vi "Transcriptor LabVIEW to C code Translator Native Functions.vi"(0 "Input":variant=variant("Function Name"=variant(string "Strip Path"), "Input Datatypes"=variant(string[] ["error", "int"]), "Inputs"=variant(string[] ["error in", "x"]), "Node refnum"=variant(refnum<vi> refnum), "Output Datatypes"=variant(string[] ["int"]), "Outputs"=variant(string[] ["a"])), 11 "error in (no error)":errorcluster) -> (4 "Output":variant=variant("Defines"=variant(string[] []), "Includes"=variant(string[] []), "Replaced Code"=variant(string "/* LabVIEW system function 'Strip Path' not found. */")), 15 "error out":errorcluster)   [LabVIEW 2014]
doc: "An example of how to create the Translator to convert the LabVIEW VIs to Arduino C code."
panel:
  out "Outputs":string[](array[string])
  out "Inputs":string[](array[string])
  out "Output Datatypes":string[](array[string])
  out "Input Datatypes":string[](array[string])
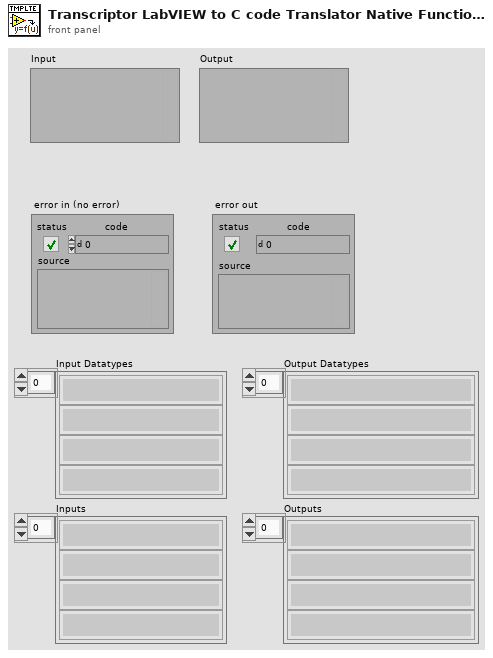
[diagram p1: front panel]
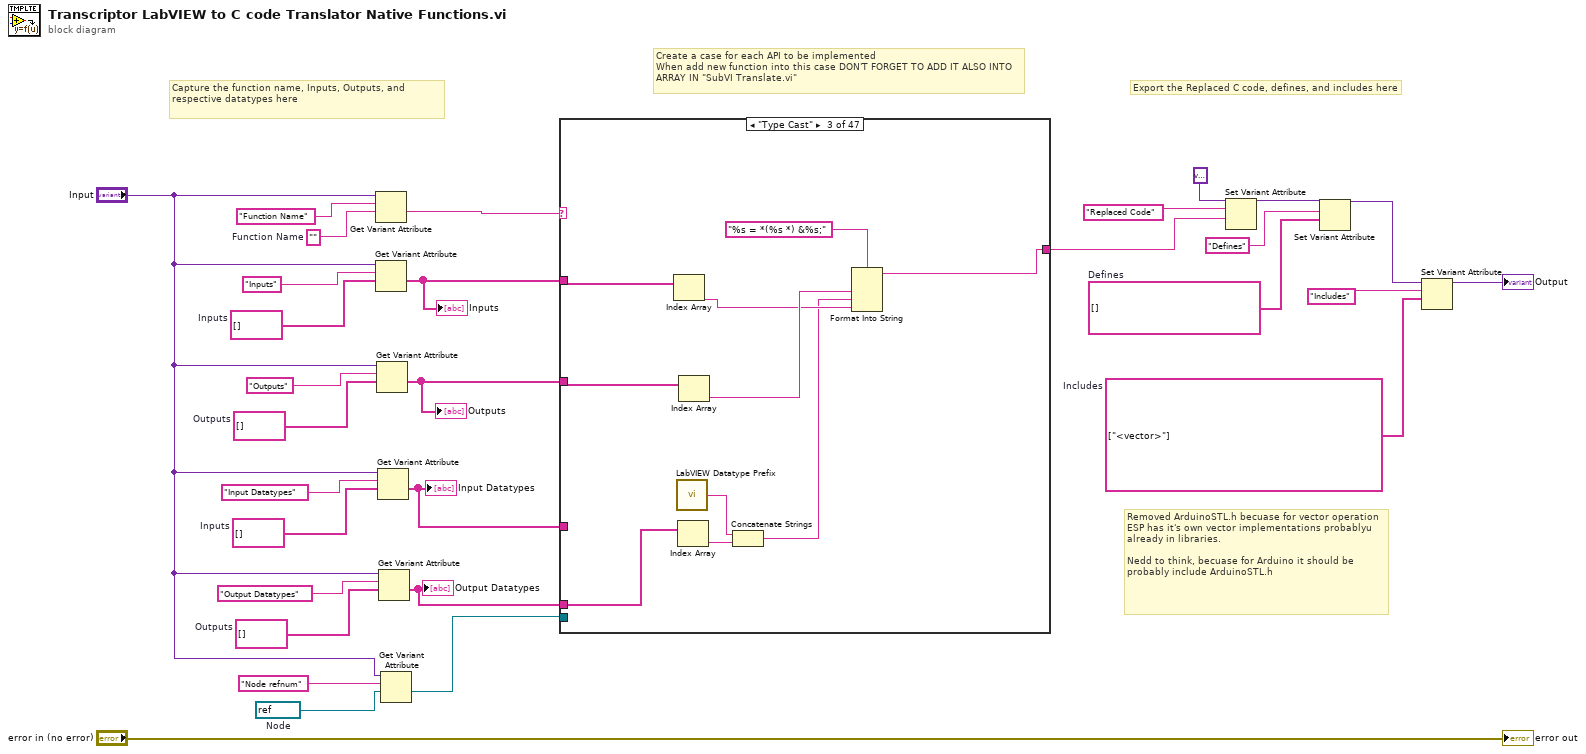
[diagram p0: block diagram]
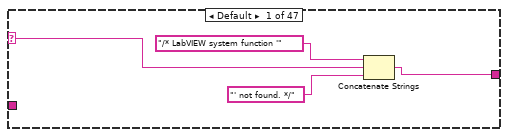
[diagram p2: hidden frame]
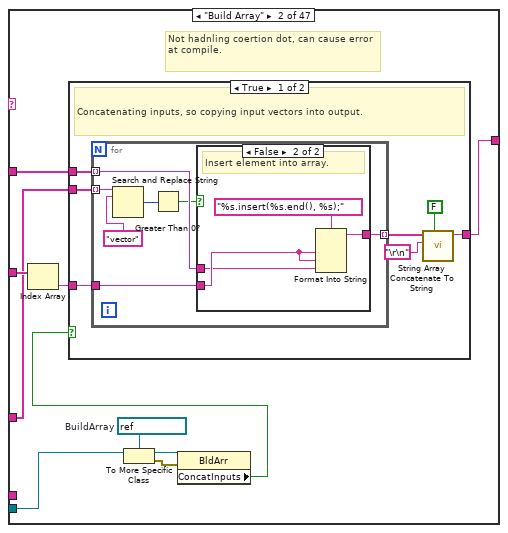
[diagram p3: hidden frame]
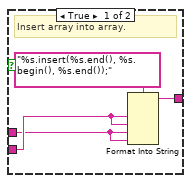
[diagram p4: hidden frame]
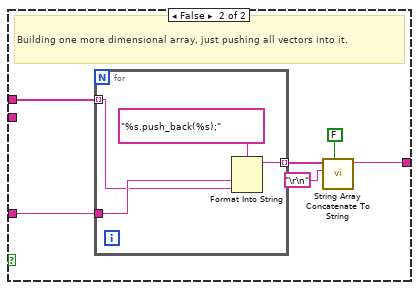
[diagram p5: hidden frame]
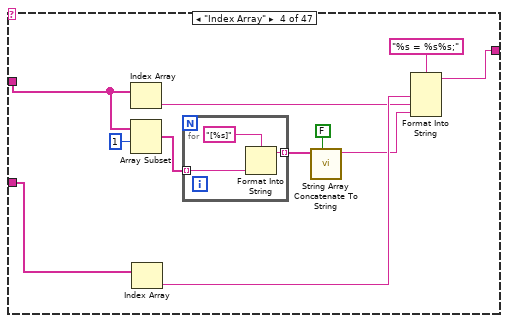
[diagram p6: hidden frame]
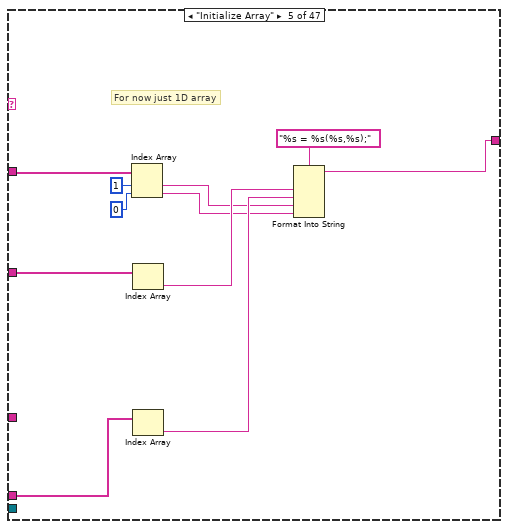
[diagram p7: hidden frame]
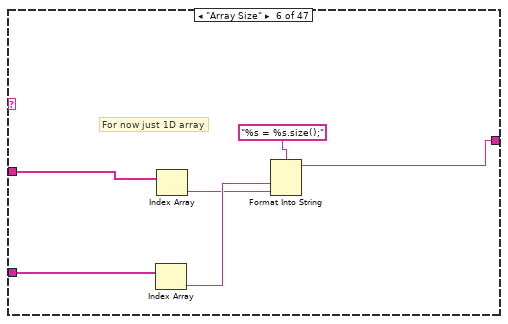
[diagram p8: hidden frame]
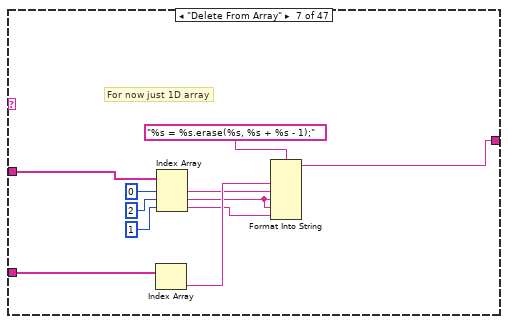
[diagram p9: hidden frame]
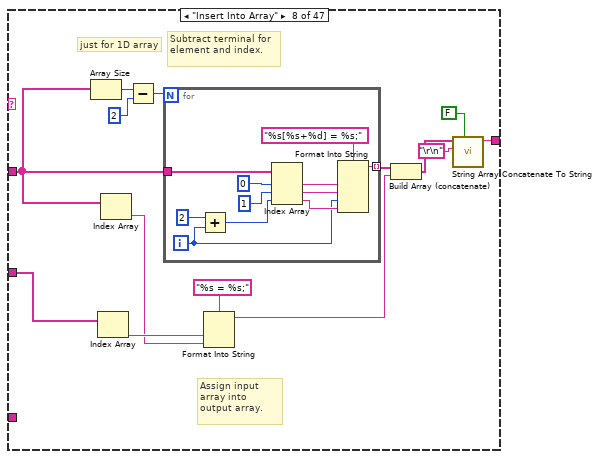
[diagram p10: hidden frame]
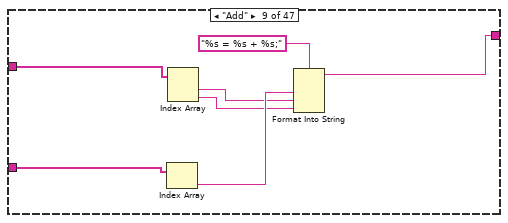
[diagram p11: hidden frame]
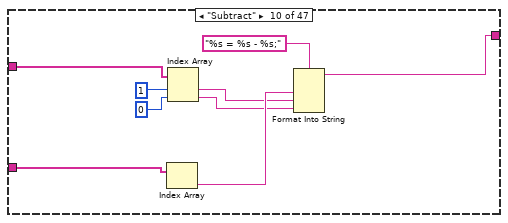
[diagram p12: hidden frame]
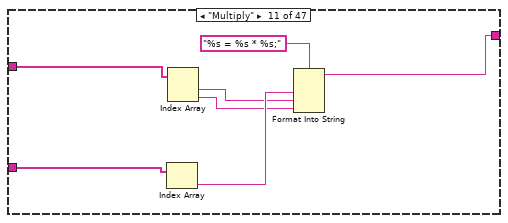
[diagram p13: hidden frame]
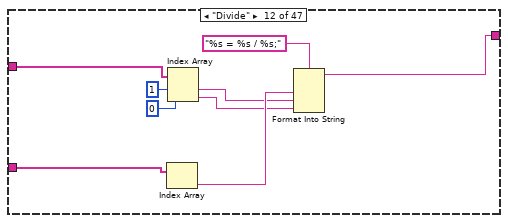
[diagram p14: hidden frame]
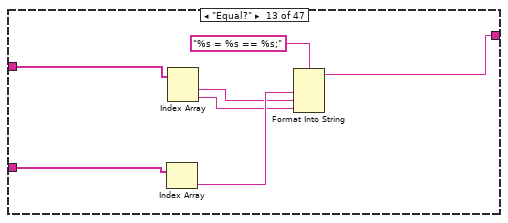
[diagram p15: hidden frame]
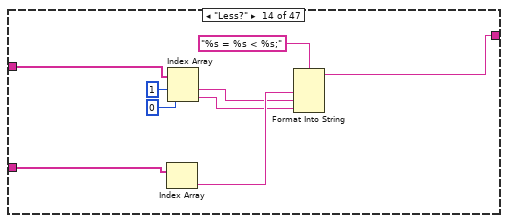
[diagram p16: hidden frame]
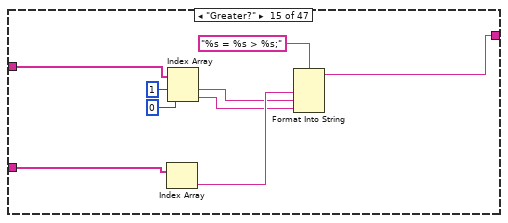
[diagram p17: hidden frame]
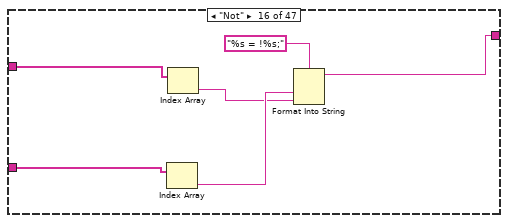
[diagram p18: hidden frame]
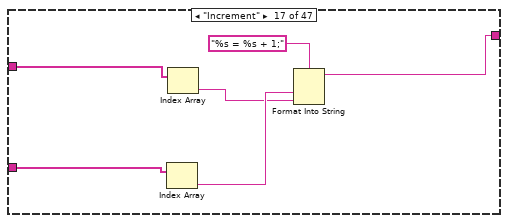
[diagram p19: hidden frame]
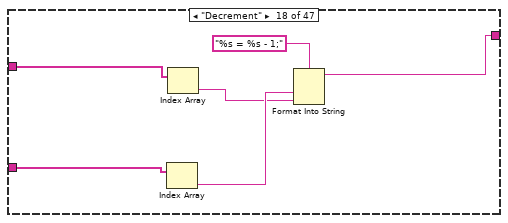
[diagram p20: hidden frame]
diagram:
  w3 = refnum<vi> refnum  # Node
  w7 = string[] []  # Defines
  w15 = string[] []  # Outputs
  w16 = string[] []  # Inputs
  w21 = string[] ["<vector>"]  # Includes
  w26 = string[] []  # Outputs
  w27 = string[] []  # Inputs
  w28 = ""  # Function Name
  # "Removed ArduinoSTL.h becuase for vector operation ESP has it's own vector implementations probablyu already in libraries.\n\nNedd to think, becuase for Arduino it should be probably include ArduinoSTL.h"
  # "Capture the function name, Inputs, Outputs, and respective datatypes here"
  # "Export the Replaced C code, defines, and includes here"
  # "Create a case for each API to be implemented\nWhen add new function into this case DON'T FORGET TO ADD IT ALSO INTO ARRAY IN \"SubVI Translate.vi\""
  n1 = Get Variant Attribute(Variant="Input", name="Function Name", default value (empty Variant)=w28) -> (value=w23:string)  [unwired: 1 in, 3 out]
  n2 = Get Variant Attribute(Variant="Input", name="Inputs", default value (empty Variant)=w27) -> (value=w12:string[])  [unwired: 1 in, 3 out]
  "Inputs" <- w12
  n3 = Get Variant Attribute(Variant="Input", name="Outputs", default value (empty Variant)=w26) -> (value=w13:string[])  [unwired: 1 in, 3 out]
  "Outputs" <- w13
  n4 = Get Variant Attribute(Variant="Input", name="Input Datatypes", default value (empty Variant)=w16) -> (value=w6:string[])  [unwired: 1 in, 3 out]
  "Input Datatypes" <- w6
  n5 = Get Variant Attribute(Variant="Input", name="Output Datatypes", default value (empty Variant)=w15) -> (value=w1:string[])  [unwired: 1 in, 3 out]
  "Output Datatypes" <- w1
  n6 = Get Variant Attribute(Variant="Input", name="Node refnum", default value (empty Variant)=w3) -> (value=w2:refnum<vi>)  [unwired: 1 in, 3 out]
  n7 = case shown="\"Type Cast\"" w23 {
    selector: w23 -> [w33 _ _ _ _ _ _ _ _ _ _ _ _ _ _ _ _ _ _ _ _ _ _ _ _ _ _ _ _ _ _ _ _ _ _ _ _ _ _ _ _ _ _ _ _ _ _]
    tunnel: [w31 w41 w85 w93 w101 w112 w123 w140 w154 w163 w170 w179 w186 w195 w204 w211 w217 w223 w229 w235 w241 w247 w253 w259 w266 w273 w280 w286 w293 w300 w307 w311 w318 w323 w338 w355 w365 w375 w385 w391 w397 w403 w409 w415 w421 w427 w433] -> w22
    tunnel: w12 -> [_ w43 w84 w92 w111 w117 w128 w133 w160 w169 w176 w185 w192 w201 w210 w216 w222 w228 w234 w240 w246 w252 w258 w265 w272 w279 w285 w292 w299 w306 w310 w314 w320 w322 w340 w352 w362 w372 w384 w390 w396 w402 w408 w414 w420 w426 w432]
    tunnel: w13 -> [_ w44 w83 w97 w110 w115 w126 w136 w158 w167 w174 w183 w190 w199 w208 w214 w220 w226 w232 w238 w244 w250 w256 w263 w270 w277 w283 w290 w297 w304 _ _ w316 w321 w339 w349 w359 w369 w380 w389 w395 w401 w407 w413 w419 w425 w431]
    tunnel: w6 -> [_ w35 _ _ _ _ _ _ _ _ _ _ _ _ _ _ _ _ _ _ _ _ _ _ _ _ _ _ _ _ _ _ _ _ _ _ _ _ _ _ _ _ _ _ _ _ _]
    tunnel: w2 -> [_ w40 _ _ _ _ _ _ _ _ _ _ _ _ _ _ _ _ _ _ _ _ _ _ _ _ _ _ _ _ _ _ _ _ _ _ _ _ _ _ _ _ _ _ _ _ _]
    tunnel: w1 -> [_ _ w77 _ w106 _ _ _ _ _ _ _ _ _ _ _ _ _ _ _ _ _ _ _ _ _ _ _ _ _ _ _ _ _ _ _ _ _ _ _ _ _ _ _ _ _ _]
    frame Default {
      n8 = Concatenate Strings("/* LabVIEW system function '", w33, "' not found. */") -> (w31:string)
    }
    frame "Build Array" {
      w39 = refnum<vi> refnum  # BuildArray
      # "Not hadnling coertion dot, can cause error at compile."
      n9 = Index Array(array=w44) -> (element=w42:string)  [unwired: 1 in]
      n10 = To More Specific Class(target class=w39, reference=w40) -> (specific class reference=w38:refnum<vi>, error out=w37:errorcluster)  [unwired: 1 in]
      n11 = property class="BldArr"(reference=w38, error in=w37) -> ("ConcatInputs"=w36:bool)  [unwired: 2 out]
      n12 = case shown="True" w36 {
        tunnel: w43 -> [w51 w72]
        tunnel: w42 -> [w50 w71]
        tunnel: [w46 w67] -> w41
        tunnel: w35 -> [w45 _]
        frame True {
          # "Concatenating inputs, so copying input vectors into output."
          n13 = for {
            tunnel: w51 -> [w57] mode=indexing
            tunnel: w50 -> [w58]
            tunnel: [w56] -> w49 mode=indexing
            tunnel: w45 -> [w55] mode=indexing
            n14 = Search and Replace String(input string=w55, search string="vector" ("name")) -> (number of replacements=w53:i32)  [unwired: 6 in, 3 out]
            n15 = Greater Than 0?(x=w53) -> (x > 0?=w52:bool)
            n16 = case shown="False" w52 {
              tunnel: w58 -> [w61 w65]
              tunnel: w57 -> [w60 w64]
              tunnel: [w59 w63] -> w56
              frame True {
                # "Insert array into array."
                n17 = Format Into String(format string="%s.insert(%s.end(), %s.begin(), %s.end());" ("name"), w61, w61, w60, w60) -> (resulting string=w59:string)  [unwired: 2 in, 1 out]
              }
              frame False {
                # "Insert element into array."
                n18 = Format Into String(format string="%s.insert(%s.end(), %s);" ("name"), w65, w65, w64) -> (resulting string=w63:string)  [unwired: 2 in, 1 out]
              }
            }
          }
          n19 = call "String Array Concatenate To String.vi"("insert last delimiter?"=FALSE, "Delimiter char"="\r\n", "Array String In"=w49) -> ("String"=w46:string)  [unwired: 8 in]
        }
        frame False {
          # "Building one more dimensional array, just pushing all vectors into it."
          n20 = for {
            tunnel: w72 -> [w74] mode=indexing
            tunnel: w71 -> [w75]
            tunnel: [w73] -> w70 mode=indexing
            n21 = Format Into String(format string="%s.push_back(%s);" ("name"), w75, w74) -> (resulting string=w73:string)  [unwired: 2 in, 1 out]
          }
          n22 = call "String Array Concatenate To String.vi"("insert last delimiter?"=FALSE, "Delimiter char"="\r\n", "Array String In"=w70) -> ("String"=w67:string)  [unwired: 8 in]
        }
      }
    }
    frame "Type Cast" {
      n23 = Index Array(array=w84) -> (element=w81:string)  [unwired: 1 in]
      n24 = call "LabVIEW Datatype Prefix.vi"() -> ("datatype prefix"=w78:string)
      n25 = Index Array(array=w77) -> (element=w80:string)  [unwired: 1 in]
      n26 = Index Array(array=w83) -> (element=w82:string)  [unwired: 1 in]
      n27 = Concatenate Strings(w78, w80) -> (w79:string)
      n28 = Format Into String(format string="%s = *(%s *) &%s;" ("name"), w82, w79, w81) -> (resulting string=w85:string)  [unwired: 2 in, 1 out]
    }
    frame "Index Array" {
      n29 = Index Array(array=w92) -> (element=w94:string)  [unwired: 1 in]
      n30 = Array Subset(array=w92, index=1) -> (w90:string[])  [unwired: 1 in]
      n31 = Index Array(array=w97) -> (element=w95:string)  [unwired: 1 in]
      n32 = for {
        tunnel: w90 -> [w99] mode=indexing
        tunnel: [w98] -> w88 mode=indexing
        n33 = Format Into String(format string="[%s]", w99) -> (resulting string=w98:string)  [unwired: 2 in, 1 out]
      }
      n34 = call "String Array Concatenate To String.vi"("insert last delimiter?"=FALSE, "Array String In"=w88) -> ("String"=w87:string)  [unwired: 9 in]
      n35 = Format Into String(format string="%s = %s%s;", w95, w94, w87) -> (resulting string=w93:string)  [unwired: 2 in, 1 out]
    }
    frame "Initialize Array" {
      # "For now just 1D array"
      n36 = Index Array(array=w111, index #1=1 ("index"), index #2=0 ("index")) -> (element #1=w103:string, element #2=w102:string)
      n37 = Index Array(array=w110) -> (element=w108:string)  [unwired: 1 in]
      n38 = Index Array(array=w106) -> (element=w107:string)  [unwired: 1 in]
      n39 = Format Into String(format string="%s = %s(%s,%s);", w108, w107, w103, w102) -> (resulting string=w101:string)  [unwired: 2 in, 1 out]
    }
    frame "Array Size" {
      # "For now just 1D array"
      n40 = Index Array(array=w115) -> (element=w114:string)  [unwired: 1 in]
      n41 = Index Array(array=w117) -> (element=w113:string)  [unwired: 1 in]
      n42 = Format Into String(format string="%s = %s.size();", w114, w113) -> (resulting string=w112:string)  [unwired: 2 in, 1 out]
    }
    frame "Delete From Array" {
      # "For now just 1D array"
      n43 = Index Array(array=w126) -> (element=w125:string)  [unwired: 1 in]
      n44 = Index Array(array=w128, index #1=0 ("index"), index #2=2 ("index"), index #3=1 ("index")) -> (element #1=w124:string, element #2=w119:string, element #3=w118:string)
      n45 = Format Into String(format string="%s = %s.erase(%s, %s + %s - 1);", w125, w124, w119, w119, w118) -> (resulting string=w123:string)  [unwired: 2 in, 1 out]
    }
    frame "Insert Into Array" {
      # "just for 1D array"
      # "Subtract terminal for element and index."
      # "Assign input array into output array."
      n46 = Array Size(array=w133) -> (size(s)=w138:i32)
      n47 = Index Array(array=w136) -> (element=w134:string)  [unwired: 1 in]
      n48 = Index Array(array=w133) -> (element=w132:string)  [unwired: 1 in]
      n49 = Subtract(x=w138, y=2) -> (x-y=w139:i32)
      n50 = for {
        N: w139 -> [_]
        tunnel: w133 -> [w150]
        tunnel: [w151] -> w131 mode=indexing
        i -> [w146]
        n51 = Add(x=2, y=w146) -> (x+y=w145:i32)
        n52 = Index Array(array=w150, index #1=0 ("index"), index #2=1 ("index"), index #3=w145) -> (element #1=w143:string, element #2=w152:string, element #3=w148:string)
        n53 = Format Into String(format string="%s[%s+%d] = %s;", w143, w152, w146, w148) -> (resulting string=w151:string)  [unwired: 2 in, 1 out]
      }
      n54 = Format Into String(format string="%s = %s;", w134, w132) -> (resulting string=w130:string)  [unwired: 2 in, 1 out]
      n55 = Build Array (concatenate)(w131, w130) -> (w129:string[])
      n56 = call "String Array Concatenate To String.vi"("insert last delimiter?"=FALSE, "Delimiter char"="\r\n", "Array String In"=w129) -> ("String"=w140:string)  [unwired: 8 in]
    }
    frame "Add" {
      n57 = Index Array(array=w158) -> (element=w157:string)  [unwired: 1 in]
      n58 = Index Array(array=w160) -> (element #1=w156:string, element #2=w155:string)  [unwired: 2 in]
      n59 = Format Into String(format string="%s = %s + %s;", w157, w156, w155) -> (resulting string=w154:string)  [unwired: 2 in, 1 out]
    }
    frame "Subtract" {
      n60 = Index Array(array=w167) -> (element=w166:string)  [unwired: 1 in]
      n61 = Index Array(array=w169, index #1=1 ("index"), index #2=0 ("index")) -> (element #1=w165:string, element #2=w164:string)
      n62 = Format Into String(format string="%s = %s - %s;", w166, w165, w164) -> (resulting string=w163:string)  [unwired: 2 in, 1 out]
    }
    frame "Multiply" {
      n63 = Index Array(array=w174) -> (element=w173:string)  [unwired: 1 in]
      n64 = Index Array(array=w176) -> (element #1=w172:string, element #2=w171:string)  [unwired: 2 in]
      n65 = Format Into String(format string="%s = %s * %s;", w173, w172, w171) -> (resulting string=w170:string)  [unwired: 2 in, 1 out]
    }
    frame "Divide" {
      n66 = Index Array(array=w183) -> (element=w182:string)  [unwired: 1 in]
      n67 = Index Array(array=w185, index #1=1 ("index"), index #2=0 ("index")) -> (element #1=w181:string, element #2=w180:string)
      n68 = Format Into String(format string="%s = %s / %s;", w182, w181, w180) -> (resulting string=w179:string)  [unwired: 2 in, 1 out]
    }
    frame "Equal?" {
      n69 = Index Array(array=w190) -> (element=w189:string)  [unwired: 1 in]
      n70 = Index Array(array=w192) -> (element #1=w188:string, element #2=w187:string)  [unwired: 2 in]
      n71 = Format Into String(format string="%s = %s == %s;", w189, w188, w187) -> (resulting string=w186:string)  [unwired: 2 in, 1 out]
    }
    frame "Less?" {
      n72 = Index Array(array=w199) -> (element=w198:string)  [unwired: 1 in]
      n73 = Index Array(array=w201, index #1=1 ("index"), index #2=0 ("index")) -> (element #1=w197:string, element #2=w196:string)
      n74 = Format Into String(format string="%s = %s < %s;", w198, w197, w196) -> (resulting string=w195:string)  [unwired: 2 in, 1 out]
    }
    frame "Greater?" {
      n75 = Index Array(array=w208) -> (element=w207:string)  [unwired: 1 in]
      n76 = Index Array(array=w210, index #1=1 ("index"), index #2=0 ("index")) -> (element #1=w206:string, element #2=w205:string)
      n77 = Format Into String(format string="%s = %s > %s;", w207, w206, w205) -> (resulting string=w204:string)  [unwired: 2 in, 1 out]
    }
    frame "Not" {
      n78 = Index Array(array=w214) -> (element=w213:string)  [unwired: 1 in]
      n79 = Index Array(array=w216) -> (element=w212:string)  [unwired: 1 in]
      n80 = Format Into String(format string="%s = !%s;", w213, w212) -> (resulting string=w211:string)  [unwired: 2 in, 1 out]
    }
    frame "Increment" {
      n81 = Index Array(array=w220) -> (element=w219:string)  [unwired: 1 in]
      n82 = Index Array(array=w222) -> (element=w218:string)  [unwired: 1 in]
      n83 = Format Into String(format string="%s = %s + 1;", w219, w218) -> (resulting string=w217:string)  [unwired: 2 in, 1 out]
    }
    frame "Decrement" {
      n84 = Index Array(array=w226) -> (element=w225:string)  [unwired: 1 in]
      n85 = Index Array(array=w228) -> (element=w224:string)  [unwired: 1 in]
      n86 = Format Into String(format string="%s = %s - 1;", w225, w224) -> (resulting string=w223:string)  [unwired: 2 in, 1 out]
    }
    frame "Equal To 0?" {
      n87 = Index Array(array=w232) -> (element=w231:string)  [unwired: 1 in]
      n88 = Index Array(array=w234) -> (element=w230:string)  [unwired: 1 in]
      n89 = Format Into String(format string="%s = (%s == 0);", w231, w230) -> (resulting string=w229:string)  [unwired: 2 in, 1 out]
    }
    frame "Greater Than 0?" {
      n90 = Index Array(array=w238) -> (element=w237:string)  [unwired: 1 in]
      n91 = Index Array(array=w240) -> (element=w236:string)  [unwired: 1 in]
      n92 = Format Into String(format string="%s = (%s > 0);", w237, w236) -> (resulting string=w235:string)  [unwired: 2 in, 1 out]
    }
    frame "Less Than 0?" {
      n93 = Index Array(array=w244) -> (element=w243:string)  [unwired: 1 in]
      n94 = Index Array(array=w246) -> (element=w242:string)  [unwired: 1 in]
      n95 = Format Into String(format string="%s = (%s < 0);", w243, w242) -> (resulting string=w241:string)  [unwired: 2 in, 1 out]
    }
    frame "Greater Or Equal To 0?" {
      n96 = Index Array(array=w250) -> (element=w249:string)  [unwired: 1 in]
      n97 = Index Array(array=w252) -> (element=w248:string)  [unwired: 1 in]
      n98 = Format Into String(format string="%s = (%s >= 0);", w249, w248) -> (resulting string=w247:string)  [unwired: 2 in, 1 out]
    }
    frame "Less Or Equal To 0?" {
      n99 = Index Array(array=w256) -> (element=w255:string)  [unwired: 1 in]
      n100 = Index Array(array=w258) -> (element=w254:string)  [unwired: 1 in]
      n101 = Format Into String(format string="%s = (%s <= 0);", w255, w254) -> (resulting string=w253:string)  [unwired: 2 in, 1 out]
    }
    frame "Greater Or Equal?" {
      n102 = Index Array(array=w263) -> (element=w262:string)  [unwired: 1 in]
      n103 = Index Array(array=w265) -> (element #1=w261:string, element #2=w260:string)  [unwired: 2 in]
      n104 = Format Into String(format string="%s = (%s >= %s);", w262, w261, w260) -> (resulting string=w259:string)  [unwired: 2 in, 1 out]
    }
    frame "Less Or Equal?" {
      n105 = Index Array(array=w270) -> (element=w269:string)  [unwired: 1 in]
      n106 = Index Array(array=w272) -> (element #1=w268:string, element #2=w267:string)  [unwired: 2 in]
      n107 = Format Into String(format string="%s = (%s <= %s);", w269, w268, w267) -> (resulting string=w266:string)  [unwired: 2 in, 1 out]
    }
    frame "Not Equal?" {
      n108 = Index Array(array=w277) -> (element=w276:string)  [unwired: 1 in]
      n109 = Index Array(array=w279) -> (element #1=w275:string, element #2=w274:string)  [unwired: 2 in]
      n110 = Format Into String(format string="%s = (%s != %s);", w276, w275, w274) -> (resulting string=w273:string)  [unwired: 2 in, 1 out]
    }
    frame "Not Equal To 0?" {
      n111 = Index Array(array=w283) -> (element=w282:string)  [unwired: 1 in]
      n112 = Index Array(array=w285) -> (element=w281:string)  [unwired: 1 in]
      n113 = Format Into String(format string="%s = (%s != 0);", w282, w281) -> (resulting string=w280:string)  [unwired: 2 in, 1 out]
    }
    frame "And" {
      n114 = Index Array(array=w290) -> (element=w289:string)  [unwired: 1 in]
      n115 = Index Array(array=w292) -> (element #1=w288:string, element #2=w287:string)  [unwired: 2 in]
      n116 = Format Into String(format string="%s = %s AND %s;", w289, w288, w287) -> (resulting string=w286:string)  [unwired: 2 in, 1 out]
    }
    frame "Or" {
      n117 = Index Array(array=w297) -> (element=w296:string)  [unwired: 1 in]
      n118 = Index Array(array=w299) -> (element #1=w295:string, element #2=w294:string)  [unwired: 2 in]
      n119 = Format Into String(format string="%s = %s OR %s;", w296, w295, w294) -> (resulting string=w293:string)  [unwired: 2 in, 1 out]
    }
    frame "Exclusive Or" {
      n120 = Index Array(array=w304) -> (element=w303:string)  [unwired: 1 in]
      n121 = Index Array(array=w306) -> (element #1=w302:string, element #2=w301:string)  [unwired: 2 in]
      n122 = Format Into String(format string="%s = %s XOR %s;", w303, w302, w301) -> (resulting string=w300:string)  [unwired: 2 in, 1 out]
    }
    frame "To Lower Case" {
      n123 = Index Array(array=w310) -> (element=w308:string)  [unwired: 1 in]
      n124 = Format Into String(format string="%s.toLowerCase();", w308) -> (resulting string=w307:string)  [unwired: 2 in, 1 out]
    }
    frame "To Upper Case" {
      n125 = Index Array(array=w314) -> (element=w312:string)  [unwired: 1 in]
      n126 = Format Into String(format string="%s.toUpperCase();", w312) -> (resulting string=w311:string)  [unwired: 2 in, 1 out]
    }
    frame "String Length" {
      n127 = Index Array(array=w316) -> (element=w315:string)  [unwired: 1 in]
      n128 = Index Array(array=w320) -> (element=w317:string)  [unwired: 1 in]
      n129 = Format Into String(format string="%s = %s.length();", w315, w317) -> (resulting string=w318:string)  [unwired: 2 in, 1 out]
    }
    frame "String Subset" {
      # "If more output wired take one with highes index.\n\nI'm interested just in index, no string outputs."
      n130 = Array Size(array=w321) -> (size(s)=w327:i32)
      n131 = Greater?(x=w327, y=1) -> (0:w328:bool)
      n132 = Index Array(array=w322, index #1=2 ("index"), index #2=1 ("index"), index #3=0 ("index")) -> (element #1=w334:string, element #2=w333:string, element #3=w331:string)
      n133 = Decrement(x=w327) -> (x-1=w325:i32)
      n134 = Select(t=w325, s=w328, f=0) -> (s? t:f=w324:i32)
      n135 = Index Array(array=w321, index=w324) -> (element=w335:string)
      n136 = Format Into String(format string="%s = %s.substring(%s,%s);", w335, w334, w333, w331) -> (resulting string=w323:string)  [unwired: 2 in, 1 out]
    }
    frame "Match Pattern" {
      n137 = Index Array(array=w340, index #1=1 ("index"), index #2=0 ("index"), index #3=2 ("index")) -> (element #1=w344:string, element #2=w345:string, element #3=w347:string)
      n138 = Index Array(array=w339) -> (element=w343:string)  [unwired: 1 in]
      n139 = Format Into String(format string="%s = %s.indexOf(%s,%s);", w343, w344, w345, w347) -> (resulting string=w338:string)  [unwired: 2 in, 1 out]
    }
    frame "Decimal String To Number" {
      # "Here we are hoping that user wired just one input and just one output."
      n140 = Array Size(array=w352) -> (size(s)=w354:i32)
      n141 = Array Size(array=w349) -> (size(s)=w351:i32)
      n142 = Decrement(x=w354) -> (x-1=w353:i32)
      n143 = Decrement(x=w351) -> (x-1=w350:i32)
      n144 = Index Array(array=w352, index=w353) -> (element=w358:string)
      n145 = Index Array(array=w349, index=w350) -> (element=w357:string)
      n146 = Format Into String(format string="%s = %s.toInt();", w357, w358) -> (resulting string=w355:string)  [unwired: 2 in, 1 out]
    }
    frame "Number To Fractional String" {
      # "NOT IMPLEMENTED PRECISION TERMINAL!"
      # "Here we are hoping that user wired just one input and just one output."
      n147 = Array Size(array=w362) -> (size(s)=w364:i32)
      n148 = Array Size(array=w359) -> (size(s)=w361:i32)
      n149 = Decrement(x=w364) -> (x-1=w363:i32)
      n150 = Decrement(x=w361) -> (x-1=w360:i32)
      n151 = Index Array(array=w362, index=w363) -> (element=w368:string)
      n152 = Index Array(array=w359, index=w360) -> (element=w367:string)
      n153 = Format Into String(format string="%s = String(%s);", w367, w368) -> (resulting string=w365:string)  [unwired: 2 in, 1 out]
    }
    frame "Fract/Exp String To Number" {
      # "Here we are hoping that user wired just one input and just one output."
      n154 = Array Size(array=w372) -> (size(s)=w374:i32)
      n155 = Array Size(array=w369) -> (size(s)=w371:i32)
      n156 = Decrement(x=w374) -> (x-1=w373:i32)
      n157 = Decrement(x=w371) -> (x-1=w370:i32)
      n158 = Index Array(array=w372, index=w373) -> (element=w378:string)
      n159 = Index Array(array=w369, index=w370) -> (element=w377:string)
      n160 = Format Into String(format string="%s = %s.toFloat();", w377, w378) -> (resulting string=w375:string)  [unwired: 2 in, 1 out]
    }
    frame "Number To Decimal String" {
      # "Here we are hoping that user wired just one input and just one output."
      n161 = Array Size(array=w384) -> (size(s)=w383:i32)
      n162 = Array Size(array=w380) -> (size(s)=w381:i32)
      n163 = Decrement(x=w383) -> (x-1=w382:i32)
      n164 = Decrement(x=w381) -> (x-1=w379:i32)
      n165 = Index Array(array=w384, index=w382) -> (element=w388:string)
      n166 = Index Array(array=w380, index=w379) -> (element=w387:string)
      n167 = Format Into String(format string="%s = String(%s);", w387, w388) -> (resulting string=w385:string)  [unwired: 2 in, 1 out]
    }
    frame "To Unsigned Long Integer" {
      n168 = Index Array(array=w390) -> (element=w394:string)  [unwired: 1 in]
      n169 = Index Array(array=w389) -> (element=w393:string)  [unwired: 1 in]
      n170 = Format Into String(format string="%s = (unsigned long) %s;", w393, w394) -> (resulting string=w391:string)  [unwired: 2 in, 1 out]
    }
    frame "To Double Precision Float" {
      n171 = Index Array(array=w396) -> (element=w400:string)  [unwired: 1 in]
      n172 = Index Array(array=w395) -> (element=w399:string)  [unwired: 1 in]
      n173 = Format Into String(format string="%s = (double) %s;", w399, w400) -> (resulting string=w397:string)  [unwired: 2 in, 1 out]
    }
    frame "To Single Precision Float" {
      n174 = Index Array(array=w402) -> (element=w406:string)  [unwired: 1 in]
      n175 = Index Array(array=w401) -> (element=w405:string)  [unwired: 1 in]
      n176 = Format Into String(format string="%s = (float) %s;", w405, w406) -> (resulting string=w403:string)  [unwired: 2 in, 1 out]
    }
    frame "To Unsigned Word Integer" {
      n177 = Index Array(array=w408) -> (element=w412:string)  [unwired: 1 in]
      n178 = Index Array(array=w407) -> (element=w411:string)  [unwired: 1 in]
      n179 = Format Into String(format string="%s = (unsigned short) %s;", w411, w412) -> (resulting string=w409:string)  [unwired: 2 in, 1 out]
    }
    frame "To Unsigned Byte Integer" {
      n180 = Index Array(array=w414) -> (element=w418:string)  [unwired: 1 in]
      n181 = Index Array(array=w413) -> (element=w417:string)  [unwired: 1 in]
      n182 = Format Into String(format string="%s = (unsigned byte) %s;", w417, w418) -> (resulting string=w415:string)  [unwired: 2 in, 1 out]
    }
    frame "To Byte Integer" {
      n183 = Index Array(array=w420) -> (element=w424:string)  [unwired: 1 in]
      n184 = Index Array(array=w419) -> (element=w423:string)  [unwired: 1 in]
      n185 = Format Into String(format string="%s = (byte) %s;", w423, w424) -> (resulting string=w421:string)  [unwired: 2 in, 1 out]
    }
    frame "To Word Integer" {
      n186 = Index Array(array=w426) -> (element=w430:string)  [unwired: 1 in]
      n187 = Index Array(array=w425) -> (element=w429:string)  [unwired: 1 in]
      n188 = Format Into String(format string="%s = (short) %s;", w429, w430) -> (resulting string=w427:string)  [unwired: 2 in, 1 out]
    }
    frame "To Long Integer" {
      n189 = Index Array(array=w432) -> (element=w436:string)  [unwired: 1 in]
      n190 = Index Array(array=w431) -> (element=w435:string)  [unwired: 1 in]
      n191 = Format Into String(format string="%s = (long) %s;", w435, w436) -> (resulting string=w433:string)  [unwired: 2 in, 1 out]
    }
  }
  n192 = Set Variant Attribute(Variant=variant ("variant"), name="Replaced Code", value=w22) -> (Variant out=w10:variant)  [unwired: 1 in, 2 out]
  n193 = Set Variant Attribute(Variant=w10, name="Defines", value=w7) -> (Variant out=w9:variant)  [unwired: 1 in, 2 out]
  n194 = Set Variant Attribute(Variant=w9, name="Includes", value=w21) -> (Variant out=→"Output":variant)  [unwired: 1 in, 2 out]
  "error out" <- "error in (no error)"
